vi "wrap.CheckNamedCluster.vi"(0 "class.GLue in":refnum<class "class.GLue.lvclass">, 11 "error in (no error)":errorcluster) -> (4 "class.GLue out":refnum<class "class.GLue.lvclass">, 6 "return":i32, 10 "Size":i32, 15 "error out":errorcluster)   [LabVIEW 2014, in "GLue.lvlib" / "class.GLue.lvclass"]
uses:
  class.GLue.lvclass
  class.GLue.lvclass/class.GLue.ctl
  Resources/GLue.dll
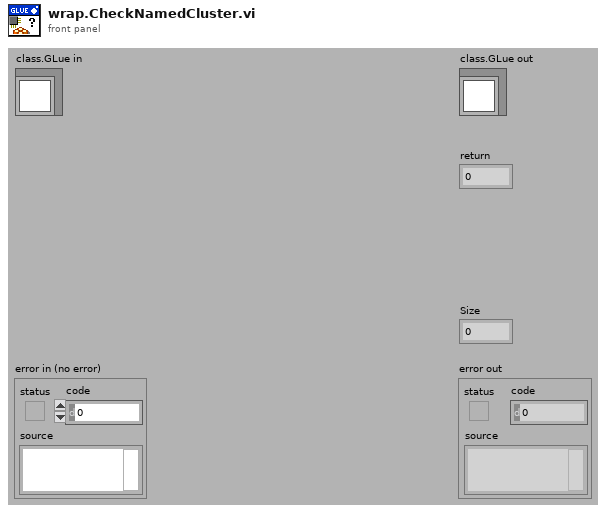
[diagram p1: front panel]
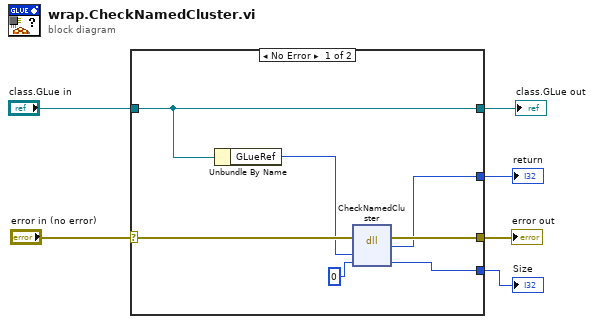
[diagram p0: block diagram]
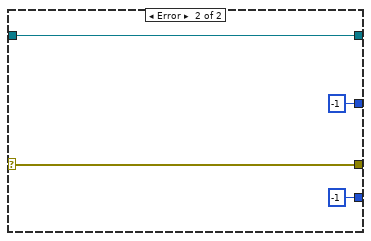
[diagram p2: hidden frame]
diagram:
  n1 = case shown="No Error" "error in (no error)" {
    selector: "error in (no error)" -> [w12 w17]
    tunnel: [w11 w17] -> w5
    tunnel: [w13 w16] -> w3
    tunnel: "class.GLue in" -> [w13 w16]
    tunnel: [w8 -1 ("Size")] -> w2
    tunnel: [w7 -1 ("return type")] -> w1
    frame No Error {
      n2 = Unbundle By Name(w13) -> ("GLueRef"=w10:i64)
      n3 = dll-call lib="C:/Users/Antonie/Documents/work/glue/trunk/Resources/GLue.dll" fn="CheckNamedCluster"(error in=w12, "MLua"=w10, "Size"=0 ("Bool")) -> (error out=w11:errorcluster, "return type"=w7:i32, "Size"=w8:i32)  [unwired: 3 in, 1 out]
    }
    frame Error {
    }
  }
  "error out" <- w5
  "class.GLue out" <- w3
  "Size" <- w2
  "return" <- w1
